vi "Launch Viewer.vi"(8 "error in (no error)":errorcluster, 11 "Application in":refnum<class "Application.lvclass">) -> (0 "error out":errorcluster, 3 "Application out":refnum<class "Application.lvclass">)   [LabVIEW 2018, in "Application.lvlib" / "Application.lvclass"]
uses:
  Application.lvclass
  C:/Program Files/National Instruments/LabVIEW 2018/vi.lib/ActorFramework/Actor/Actor.lvclass
  User Interface/Viewer/Viewer.lvclass
  C:/FlashGordon/Development/User Interface/UI Window/UI Window.lvclass
  Application.lvclass/Application.ctl
  Resources/GLOBAL/GLOBAL Time-critical.vi
  <vilib>/ActorFramework/Actor/Actor.lvclass
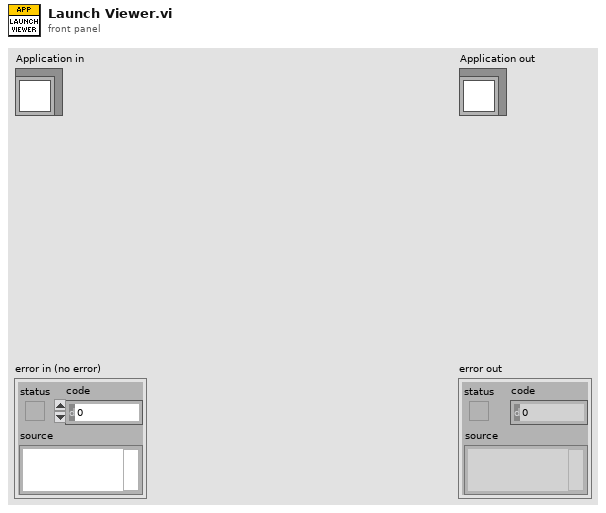
[diagram p1: front panel]
types:
  T1 = typedef "Physical Camera Assignment.ctl" = cluster{"Channel Name":string, "Camera Type":T2, "Serial Number":string, "Flip Vertically":bool, "Flip Horizontally":bool, "photonsPerCount":dbl, "wavelength":i16}
  T2 = typedef "Camera Type.ctl" = enum16{"Hamamatsu"}
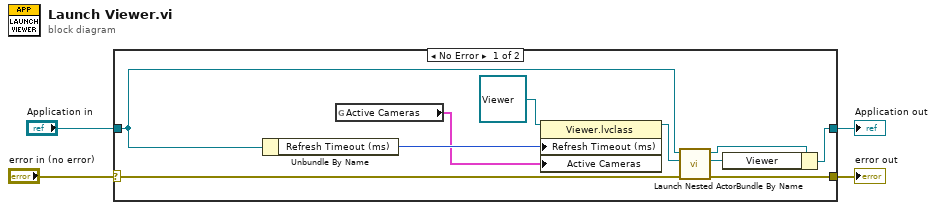
[diagram p0: block diagram]
diagram:
  n1 = case shown="No Error" "error in (no error)" {
    selector: "error in (no error)" -> [w12 w16]
    tunnel: [w11 w16] -> w3
    tunnel: [w14 w15] -> w1
    tunnel: "Application in" -> [w7 w15]
    frame No Error {
      n2 = Unbundle By Name(w7) -> ("Refresh Timeout (ms)"=w6:i32)
      n3 = global read "GLOBAL Time-critical.vi" "Active Cameras"() -> (w5:T1[])
      n4 = property class="Viewer.lvclass"(reference=refnum<class "Viewer.lvclass"> refnum ("Viewer.lvlib:Viewer.lvclass"), "Refresh Timeout (ms)"=w6, "Active Cameras"=w5) -> (reference out=w9:refnum<class "Viewer.lvclass">)  [unwired: 1 in, 1 out]
      n5 = call <vilib>:"Launch Nested Actor.vi"("error in (no error)"=w12, "Nested Actor"=w9, "Caller Actor in"=w7) -> ("error out"=w11:errorcluster, "Nested Actor's Enqueuer"=w13:refnum<class "Message Enqueuer.lvclass">, "Caller Actor out"=w8:refnum<class "Application.lvclass">)  [unwired: 6 in]
      n6 = Bundle By Name(cluster=w8, "Viewer"=w13) -> (w14:refnum<class "Application.lvclass">)
    }
    frame Error {
    }
  }
  "error out" <- w3
  "Application out" <- w1
